vi "TempodeEspera.vi"(8 "error in (no error)":errorcluster, 10 "Limite Inferior (ms)":dbl, 11 "Limite Superior (ms)":dbl) -> (0 "error out":errorcluster)   [LabVIEW 2011]
doc: "Esse VI recebe um limite de tempo inferior e um superior e realiza um sorteio de um tempo de espera dentro destes limites."
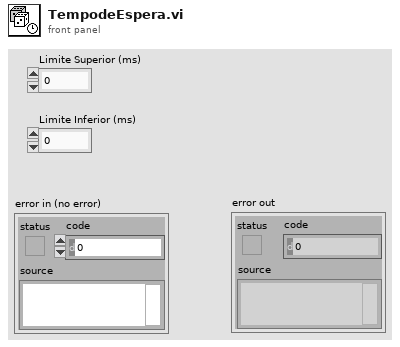
[diagram p1: front panel]
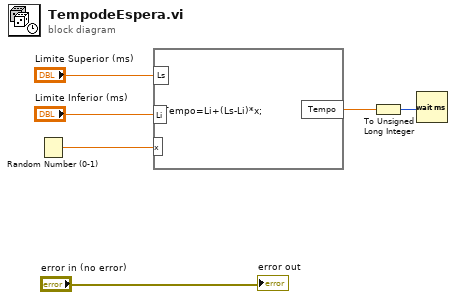
[diagram p0: block diagram]
diagram:
  n1 = Random Number (0-1)() -> (number: 0 to 1=w4:dbl)
  n2 = formula code="Tempo=Li+(Ls-Li)*x;"("Ls"="Limite Superior (ms)", "Li"="Limite Inferior (ms)", "x"=w4) -> ("Tempo"=w3:dbl)
  n3 = To Unsigned Long Integer(number=w3) -> (unsigned 32bit integer=w2:u32)
  n4 = Wait (ms)(milliseconds to wait=w2) -> ()  [unwired: 1 out]
  "error out" <- "error in (no error)"
